vi "NI 9226 Getting Started (FPGA).vi"() -> ()   [LabVIEW 2018]
doc: "This VI will continually read single point values from 4 channels of an analog input module at a specified rate."
uses:
  <vilib>/LabVIEW Targets/FPGA/cRIO/shared/nicrio_ModuleControls/nicrio_cRIO-9217_ConversionTime.ctl
  <vilib>/rvi/Emulation/niFpgaGetClockAttributes.vi
  <vilib>/rvi/Emulation/niFpgaSctlEmulationGetInTimedLoop.vi
  <vilib>/rvi/Emulation/niFpgaEmulationReportErrorSimple.vi
  <vilib>/rvi/eio/common/nirviEmuTemplatePropertySet_errors.vi
  <vilib>/rvi/eio/common/nirviEmuTemplateMethod_errors.vi
  <vilib>/rvi/Emulation/niFpgaCriticalErrorInLSC.vi
  <vilib>/eio/EIOPropertyNode/EIOPropertyNode.xnode
  <vilib>/eio/EIONode/EIONode.xnode
  <vilib>/rvi/eio/common/nirviEmuTemplatePropertyGet_errors.vi
  <vilib>/rvi/eio/common/nirviEmuTemplatePropertyGet_noerrors.vi
  <vilib>/rvi/eio/common/nirviEmuTemplatePropertySet_noerrors.vi
panel:
  out "RTD 9226 Ohms":T1 {"RTD5 RTD72" format="%.18g"; "RTD5 RTD6" format="%.18g"; "RTD5 3" format="%.18g"; "RTD4 2" format="%.18g"; "RTD0" format="%.18g"; "RTD1" format="%.18g"; "RTD2" format="%.18g"; "RTD3" format="%.18g"}
  in  "Update Configuration":bool
  in  "Conversion Time":T2
  in  "stop":bool
  out "FPGA Error Out":errorcluster
  # "Overview: Demonstrates how to acquire and scale the data from the NI 9226\nRequirements: LabVIEW Full Development System, LV FPGA, and NI RIO\nInstructions: \n1. Run NI 9226 Getting Started (Host).vi"
  # "Input Parameters"
  # "Output Parameters"
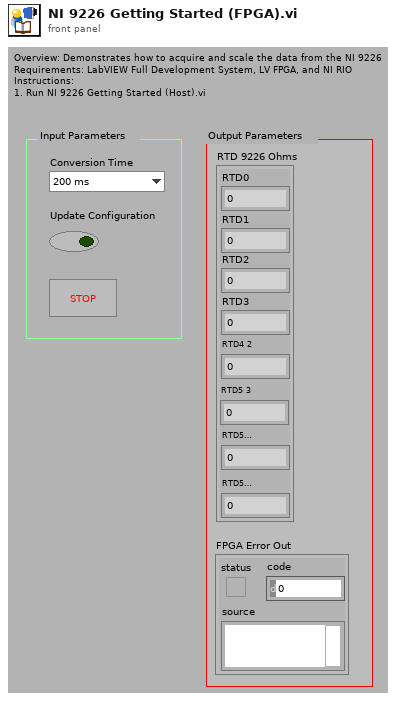
[diagram p1: front panel]
types:
  T1 = cluster{"Mod6/RTD0":fxp<+/-,24,14>, "Mod6/RTD1":fxp<+/-,24,14>, "Mod6/RTD2":fxp<+/-,24,14>, "Mod6/RTD3":fxp<+/-,24,14>, "Mod6/RTD4":fxp<+/-,24,14>, "Mod6/RTD5":fxp<+/-,24,14>, "Mod6/RTD6":fxp<+/-,24,14>, "Mod6/RTD7":fxp<+/-,24,14>}
  T2 = typedef "nicrio_cRIO-9217_ConversionTime.ctl" = enum8{"200 ms", "2.5 ms"}
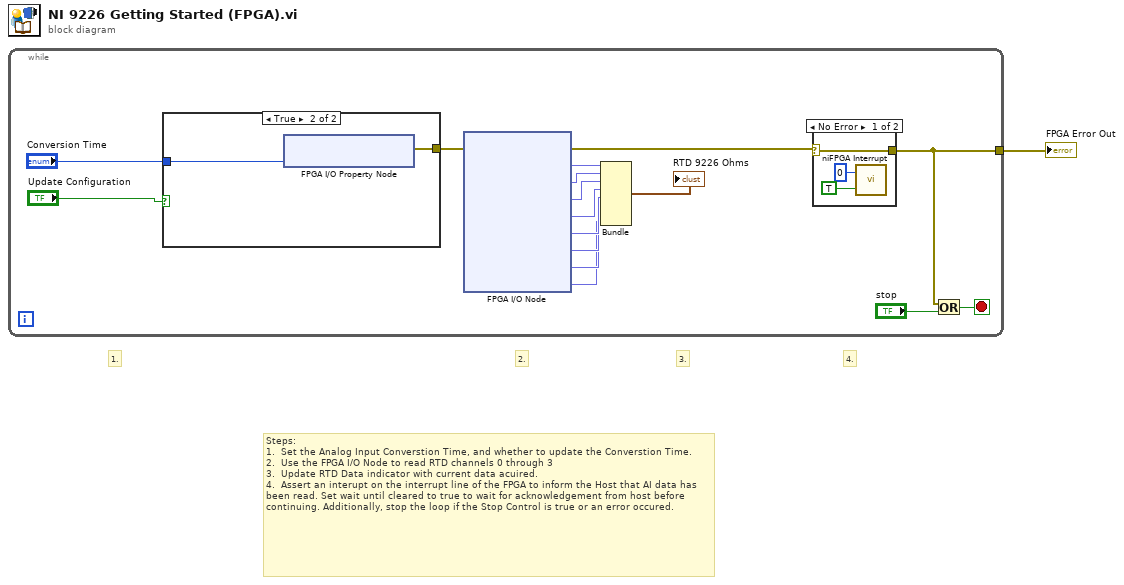
[diagram p0: block diagram]
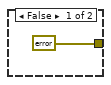
[diagram p2: hidden frame]
diagram:
  # "3."
  # "4."
  # "2."
  # "1."
  # "Steps: \n1.  Set the Analog Input Converstion Time, and whether to update the Converstion Time. \n2.  Use the FPGA I/O Node to read RTD channels 0 through 3\n3.  Update RTD Data indicator with current data acuired.\n4.  Assert an interupt on the interrupt line of the FPGA to inform the Host that AI data has been read. Set wait until cleared to true to wait for acknowledgement from host before continuing. Additionally, stop the loop if the Stop Control is true or an error occured."
  n1 = while {
    tunnel: [w15] -> w1
    stop <- w14 stop-if-true
    n2 = case shown="True" "Update Configuration" {
      tunnel: [errorcluster {"status"=FALSE, "code"=0, "source"=""} ("error out") w20] -> w7
      tunnel: "Conversion Time" -> [_ w19]
      frame False {
      }
      frame True {
        n3 = xnode "FPGA I/O Property Node"("Conversion Time"=w19) -> ("error out"=w20:errorcluster)  [unwired: 2 in, 1 out]
      }
    }
    n4 = xnode "FPGA I/O Node"("error in"=w7) -> ("error out"=w17:errorcluster, "Mod6/RTD0"=w11:fxp<+/-,24,14>, "Mod6/RTD1"=w10:fxp<+/-,24,14>, "Mod6/RTD2"=w9:fxp<+/-,24,14>, "Mod6/RTD3"=w8:fxp<+/-,24,14>, "Mod6/RTD4"=w5:fxp<+/-,24,14>, "Mod6/RTD5"=w4:fxp<+/-,24,14>, "Mod6/RTD6"=w3:fxp<+/-,24,14>, "Mod6/RTD7"=w2:fxp<+/-,24,14>)  [unwired: 8 in, 8 out]
    n5 = Bundle("Mod6/RTD0"=w11, "Mod6/RTD1"=w10, "Mod6/RTD2"=w9, "Mod6/RTD3"=w8, "Mod6/RTD4"=w5, "Mod6/RTD5"=w4, "Mod6/RTD6"=w3, "Mod6/RTD7"=w2) -> (→"RTD 9226 Ohms":T1)  [unwired: 1 out]
    n6 = case shown="No Error" w17 {
      selector: w17 -> [w21 w24]
      tunnel: [w21 w24] -> w15
      frame No Error {
        n7 = call <vilib>:"niFPGA Interrupt.vi"("Wait Until Cleared (F)"=TRUE ("Wait Until Cleared"), "IRQ Number (0)"=u8 0 ("IRQ Bit (0-31)")) -> ()  [unwired: 1 in]
      }
      frame Error {
      }
    }
    n8 = Or(x=w15, y="stop") -> (x .or. y?=w14:bool)
  }
  "FPGA Error Out" <- w1
